vi "Choreo_Trajectory_Sample.vi"(9 "MirrorForRedAlliance":bool, 10 "TimeStamp":dbl, 11 "ChoreoTrajectory":T2) -> (3 "ChoreoTrajectoryState":T1)   [LabVIEW 2019, in "ChoreoLib.lvlib"]
doc: "Return an interpolated sample of the trajectory at the given timestamp.\n\nInputs: \n - ChoreoTrajectory - cluster - The trajectory to sample.\n - timestamp - double - The timestamp of this sample relative to the beginning of the trajectory.\n - mirrorForRedAlliance - boolean - whether or not to return the sample as mirrored across the field midline (as in 2023). (Optional. Default: false )\n\nOutputs:\n - ChoreoTrajectoryState - cluster - The ChoreoTrajectoryState at the given time."
uses:
  ChoreoLib.lvlib
  TypeDef/ChoreoTrajectory.ctl
  TypeDef/ChoreoTrajectoryState.ctl
  Choreo_TrajectoryState_New.vi
  Choreo_TrajectoryState_GetAll.vi
  Choreo_TrajectoryState_FieldWidth.vi
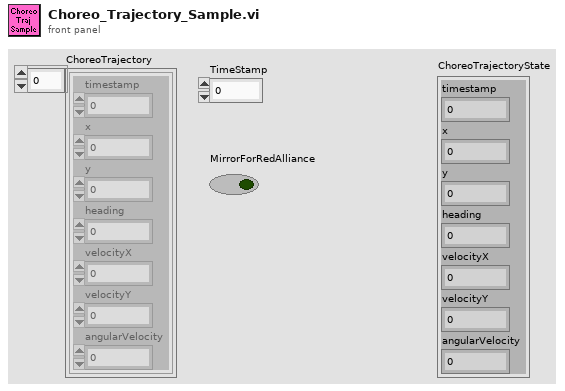
[diagram p1: front panel]
types:
  T1 = typedef "ChoreoLib.lvlib/ChoreoTrajectoryState.ctl" = cluster{"timestamp":dbl, "x":dbl, "y":dbl, "heading":dbl, "velocityX":dbl, "velocityY":dbl, "angularVelocity":dbl}
  T2 = typedef "ChoreoLib.lvlib/ChoreoTrajectory.ctl" = T1[]
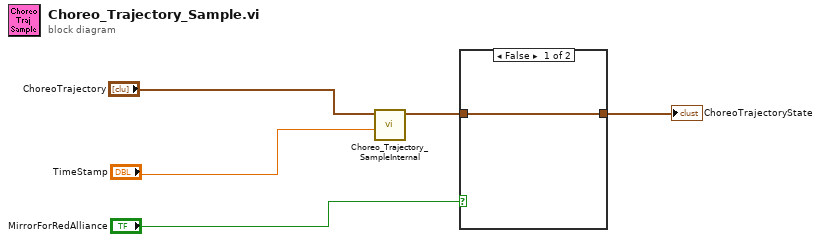
[diagram p0: block diagram]
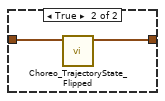
[diagram p2: hidden frame]
diagram:
  n1 = call "Choreo_Trajectory_SampleInternal.vi"("TimeStamp"="TimeStamp", "ChoreoTrajectory"="ChoreoTrajectory") -> ("ChoreoTrajectoryState"=w2:T1)  [unwired: 9 in]
  n2 = case shown="False" "MirrorForRedAlliance" {
    tunnel: w2 -> [w6 w8]
    tunnel: [w6 w7] -> w1
    frame False {
    }
    frame True {
      n3 = call "Choreo_TrajectoryState_Flipped.vi"("ChoreoTrajectoryState"=w8) -> ("flipped ChoreoTrajectoryState"=w7:T1)  [unwired: 10 in]
    }
  }
  "ChoreoTrajectoryState" <- w1
